vi "Find Repeating Ortho-Subset in GB 2014-12-15.vi"(6 "Presorted?":bool, 8 "Tolerance (A)":dbl=0.5, 9 "Slab Y":dbl=6.0, 10 "Slab X":dbl=6.0, 11 "Grain Boundary":T1={"Structure Name"="CdTe Expanded to Box", "Lattice vector a"=[19.0, 0.0, 0.0], "Lattice vector b"=[0.0, 90.0, 0.0], "Lattice vector c"=[0.0, 0.0, 19.98181818181818], "Atoms Array"=[{"Atom Name"="Cd", "Positions (Direct)"=array501x3[1503 elements], "Positions (Cartesian)"=array501x3[1503 elements]}, {"Atom Name"="Te", "Positions (Direct)"=array504x3[1512 elements], "Positions (Cartesian)"=array504x3[1512 elements]}], "# of atoms"=1005} {"Atoms Array"."Positions (Cartesian)" format="%#_4f"; "Atoms Array"."Positions (Direct)" format="%#_4f"}) -> (0 "Repeating Y Length Scale":dbl=4.670554880088597, 1 "Subset Y found?!":bool, 2 "Repeating X Length Scale":dbl, 3 "Subset X found?!":bool)   [LabVIEW 2010]
uses:
  <vilib>/Analysis/NI_AALPro.lvlib
  <vilib>/Analysis/_algsub.llb/Real Vector Norm.vi
panel:
  out "Array 3":dbl[](array[numeric])
  out "Array 2":dbl[][](array[numeric])
  out "Array":dbl[][](array[numeric])
  out "array w/ subset deleted":dbl[](array[numeric])
  in  "Y index to Search":i32=1
  in  "X index to Search":i32
  out "Length Candidates X":dbl[](array[numeric])=[0.0, 6.615785553057252, 13.231571106114504]
  out "Length Candidates Y":dbl[](array[numeric])=[4.670554880088597, 84.3349903964902, 0.0, 79.6644355164016, -4.670554880088597, 74.993880636313, 70.32332575622439, 65.6527708761358, 60.98221599604721, 56.311661115958614]
  out "Slab":T2(array[cluster])=[{"Atom Name"="Cd", "Positions (Cartesian)"=[[0.0, 4.670554880088597, 0.7469022070093141], [0.0, 0.0, 1.0119047619047619], [0.0, 4.935557434984045, 5.417457087097911], [0.0, 0.2650025548954482, 5.6824596419933595], [0.0, 5.200559989879494, 10.088011967186508], [0.0, 0.5300051097908964, 10.353014522081956], [0.0, 5.465562544774942, 14.758566847275105], [0.0, 0.7950076646863447, 15.023569402170553], [0.0, 5.73056509967039, 19.4291217273637], [0.0, 1.0600102195817929, 19.69412428225915], [3.307892776528626, 2.4677787174920227, 3.2146809245013364], [3.307892776528626, 2.732781272387471, 7.885235804589934], [3.307892776528626, 2.997783827282919, 12.55579068467853], [3.307892776528626, 3.2627863821783674, 17.226345564767126]]}, {"Atom Name"="Te", "Positions (Cartesian)"=[[1.653946388264313, 4.803056157536321, 3.0821796470536116], [1.653946388264313, 0.1325012774477241, 3.3471822019490607], [1.653946388264313, 5.068058712431769, 7.752734527142209], [1.653946388264313, 0.397503832343172, 8.017737082037657], [1.653946388264313, 5.333061267327217, 12.423289407230806], [1.653946388264313, 0.6625063872386205, 12.688291962126254], [1.653946388264313, 5.598063822222666, 17.093844287319403], [1.653946388264313, 0.9275089421340684, 17.358846842214852], [4.96183916479294, 2.3352774400442984, 0.879403484457038], [4.96183916479294, 2.6002799949397466, 5.549958364545636], [4.96183916479294, 2.865282549835195, 10.220513244634233], [4.96183916479294, 3.130285104730643, 14.891068124722828], [4.96183916479294, 3.3952876596260912, 19.561623004811427]]}] {"Positions (Cartesian)" format="%#_4f"}
  out "Supercell without slab":T2(array[cluster])=[{"Atom Name"="Cd", "Positions (Cartesian)"=[0.0, 14.01166464026579, 0.21689709721841766, 0.0, 9.341109760177194, 0.48189965211386543, 0.0, 89.0055452765788, 0.6474110989798403, 0.0, 4.670554880088597, 0.7469022070093141, 0.0, 84.3349903964902, 0.9124136538752889, 0.0, 0.0, 1.0119047619047619, 0.0, 79.6644355164016, 1.1774162087707394, 0.0, 74.993880636313, 1.442418763666188, 0.0, 70.3233257562244, 1.7074213185616385, 0.0, 65.6527708761358, 1.9724238734570871, 0.0, 60.98221599604721, 2.2374264283525305, 0.0, 56.311661115958614, 2.502428983247979, 0.0, 51.64110623587002, 2.7674315381434296, 0.0, 46.97055135578142, 3.0324340930388782, 0.0, 42.29999647569282, 3.297436647934325, 0.0, 37.62944159560422, 3.5624392028297738, 0.0, 32.95888671551563, 3.8274417577252207, 0.0, 28.288331835427034, 4.092444312620669, 0.0, 23.617776955338435, 4.357446867516118, 0.0, 18.947222075249837, 4.622449422411567, 0.0, 14.27666719516124, 4.887451977307014, 0.0, 9.606112315072641, 5.152454532202463, 0.0, 89.27054783147425, 5.317965979068438, 0.0, 4.935557434984045, 5.417457087097911, 0.0, 84.59999295138564, 5.582968533963888, 0.0, 0.2650025548954482, 5.6824596419933595, 0.0, 79.92943807129704, 5.847971088859337, 0.0, 75.25888319120845, 6.1129736437547875, 0.0, 70.58832831111985, 6.377976198650236, 0.0, 65.91777343103126, 6.6429787535456795, 0.0, 61.247218550942655, 6.907981308441128, 0.0, 56.57666367085406, 7.172983863336579, 0.0, 51.906108790765465, 7.437986418232027, 0.0, 47.23555391067687, 7.702988973127474, 0.0, 42.56499903058827, 7.967991528022923, 0.0, 37.89444415049967, 8.23299408291837, 0.0, 33.22388927041108, 8.497996637813818, 0.0, 28.55333439032248, 8.762999192709266, 0.0, 23.882779510233885, 9.028001747604716, 0.0, 19.212224630145286, 9.293004302500165, 0.0, 14.541669750056688, 9.558006857395611, 0.0, 9.87111486996809, 9.82300941229106, 0.0, 89.53555038636969, 9.988520859157038, 0.0, 5.200559989879494, 10.088011967186508, 0.0, 84.86499550628109, 10.253523414052486, 0.0, 0.5300051097908964, 10.353014522081956, 0.0, 80.19444062619249, 10.518525968947937, 0.0, 75.5238857461039, 10.783528523843385, 0.0, 70.85333086601531, 11.04853107873883, 0.0, 66.18277598592671, 11.313533633634277, 0.0, 61.51222110583811, 11.578536188529728, 0.0, 56.841666225749506, 11.843538743425176, 0.0, 52.17111134566091, 12.108541298320624, 0.0, 47.500556465572316, 12.373543853216072, 0.0, 42.83000158548372, 12.63854640811152, 0.0, 38.15944670539512, 12.903548963006967, 0.0, 33.488891825306524, 13.168551517902415, 0.0, 28.81833694521793, 13.433554072797865, 0.0, 24.14778206512933, 13.698556627693314, 0.0, 19.477227185040736, 13.963559182588762, 0.0, 14.806672304952137, 14.22856173748421, 0.0, 10.136117424863539, 14.493564292379657, 0.0, 89.80055294126514, 14.659075739245635, 0.0, 5.465562544774942, 14.758566847275105, 0.0, 85.12999806117654, 14.924078294141086, 0.0, 0.7950076646863447, 15.023569402170553, 0.0, 80.45944318108793, 15.189080849036534, 0.0, 75.78888830099935, 15.454083403931978, 0.0, 71.11833342091076, 15.719085958827426, 0.0, 66.44777854082216, 15.984088513722877, 0.0, 61.777223660733554, 16.249091068618327, 0.0, 57.10666878064496, 16.514093623513773, 0.0, 52.43611390055636, 16.77909617840922, 0.0, 47.76555902046776, 17.04409873330467, 0.0, 43.09500414037917, 17.309101288200118, 0.0, 38.42444926029057, 17.574103843095568, 0.0, 33.75389438020197, 17.839106397991014, 0.0, 29.083339500113375, 18.104108952886463, 0.0, 24.41278462002478, 18.36911150778191, 0.0, 19.74222973993618, 18.63411406267736, 0.0, 15.071674859847585, 18.89911661757281, 0.0, 10.401119979758988, 19.164119172468254, 0.0, 5.73056509967039, 19.4291217273637, 0.0, 85.39500061607198, 19.594633174229685, 0.0, 1.0600102195817929, 19.69412428225915, 0.0, 80.7244457359834, 19.859635729125127, 3.307892776528626, 58.51443727855519, 0.03465026575595598, 3.307892776528626, 53.84388239846659, 0.2996528206514042, 3.307892776528626, 49.173327518377995, 0.5646553755468551, 3.307892776528626, 44.5027726382894, 0.8296579304423033, 3.307892776528626, 39.8322177582008, 1.0946604853377506, 3.307892776528626, 35.161662878112196, 1.3596630402331988, 3.307892776528626, 30.491107998023608, 1.6246655951286462, 3.307892776528626, 25.82055311793501, 1.8896681500240944, 3.307892776528626, 21.14999823784641, 2.1546707049195435, 3.307892776528626, 16.479443357757813, 2.4196732598149917, 3.307892776528626, 11.808888477669216, 2.68467581471044, 3.307892776528626, 7.138333597580619, 2.949678369605888, 3.307892776528626, 86.80276911398222, 3.115189816471863, 3.307892776528626, 2.4677787174920227, 3.2146809245013364, 3.307892776528626, 82.13221423389362, 3.380192371367314, 3.307892776528626, 77.46165935380502, 3.645194926262762, 3.307892776528626, 72.79110447371643, 3.910197481158213, 3.307892776528626, 68.12054959362783, 4.175200036053662, 3.307892776528626, 63.44999471353923, 4.440202590949105, 3.307892776528626, 58.77943983345064, 4.705205145844554, 3.307892776528626, 54.10888495336204, 4.970207700740004, 3.307892776528626, 49.43833007327345, 5.235210255635453, 3.307892776528626, 44.767775193184846, 5.5002128105309, 3.307892776528626, 40.097220313096244, 5.765215365426348, 3.307892776528626, 35.426665433007656, 6.030217920321795, 3.307892776528626, 30.756110552919058, 6.295220475217244, 3.307892776528626, 26.08555567283046, 6.5602230301126925, 3.307892776528626, 21.41500079274186, 6.825225585008141, 3.307892776528626, 16.744445912653262, 7.090228139903589, 3.307892776528626, 12.073891032564665, 7.355230694799037, 3.307892776528626, 7.403336152476069, 7.620233249694485, 3.307892776528626, 87.06777166887767, 7.785744696560463, 3.307892776528626, 2.732781272387471, 7.885235804589934, 3.307892776528626, 82.39721678878907, 8.050747251455912, 3.307892776528626, 77.72666190870048, 8.315749806351363, 3.307892776528626, 73.05610702861188, 8.58075236124681, 3.307892776528626, 68.38555214852329, 8.845754916142255, 3.307892776528626, 63.714997268434686, 9.110757471037703, 3.307892776528626, 59.044442388346084, 9.375760025933154, 3.307892776528626, 54.37388750825748, 9.640762580828602, 3.307892776528626, 49.703332628168894, 9.90576513572405, 3.307892776528626, 45.03277774808029, 10.170767690619497, 3.307892776528626, 40.3622228679917, 10.435770245514945, 3.307892776528626, 35.6916679879031, 10.700772800410393, 3.307892776528626, 31.021113107814504, 10.96577535530584, 3.307892776528626, 26.350558227725905, 11.23077791020129, 3.307892776528626, 21.68000334763731, 11.49578046509674, 3.307892776528626, 17.00944846754871, 11.760783019992187, 3.307892776528626, 12.338893587460113, 12.025785574887635, 3.307892776528626, 7.668338707371516, 12.290788129783083, 3.307892776528626, 87.33277422377311, 12.45629957664906, 3.307892776528626, 2.997783827282919, 12.55579068467853, 3.307892776528626, 82.66221934368451, 12.721302131544512, 3.307892776528626, 77.99166446359591, 12.98630468643996, 3.307892776528626, 73.32110958350734, 13.251307241335404, 3.307892776528626, 68.65055470341873, 13.516309796230852, 3.307892776528626, 63.97999982333013, 13.781312351126303, 3.307892776528626, 59.30944494324153, 14.04631490602175, 3.307892776528626, 54.638890063152935, 14.311317460917198, 3.307892776528626, 49.96833518306434, 14.576320015812646, 3.307892776528626, 45.297780302975745, 14.841322570708094, 3.307892776528626, 40.62722542288715, 15.106325125603542, 3.307892776528626, 35.95667054279855, 15.37132768049899, 3.307892776528626, 31.28611566270995, 15.63633023539444, 3.307892776528626, 26.615560782621355, 15.901332790289889, 3.307892776528626, 21.945005902532756, 16.166335345185335, 3.307892776528626, 17.27445102244416, 16.431337900080784, 3.307892776528626, 12.603896142355563, 16.69634045497623, 3.307892776528626, 7.933341262266964, 16.96134300987168, 3.307892776528626, 87.59777677866856, 17.12685445673766, 3.307892776528626, 3.2627863821783674, 17.226345564767126, 3.307892776528626, 82.92722189857996, 17.391857011633107, 3.307892776528626, 78.25666701849137, 17.656859566528553, 3.307892776528626, 73.58611213840277, 17.921862121424, 3.307892776528626, 68.91555725831418, 18.186864676319452, 3.307892776528626, 64.24500237822558, 18.451867231214898, 3.307892776528626, 59.57444749813698, 18.716869786110347, 3.307892776528626, 54.90389261804839, 18.981872341005793, 3.307892776528626, 50.233337737959786, 19.246874895901243, 3.307892776528626, 45.562782857871184, 19.51187745079669, 3.307892776528626, 40.892227977782596, 19.776880005692142, 6.615785553057252, 14.01166464026579, 0.21689709721841766, 6.615785553057252, 9.341109760177194, 0.48189965211386543, 6.615785553057252, 89.0055452765788, 0.6474110989798403, 6.615785553057252, 4.670554880088597, 0.7469022070093141, 6.615785553057252, 84.3349903964902, 0.9124136538752889, 6.615785553057252, 0.0, 1.0119047619047619, 6.615785553057252, 79.6644355164016, 1.1774162087707394, 6.615785553057252, 74.993880636313, 1.442418763666188, 6.615785553057252, 70.3233257562244, 1.7074213185616385, 6.615785553057252, 65.6527708761358, 1.9724238734570871, 6.615785553057252, 60.98221599604721, 2.2374264283525305, 6.615785553057252, 56.311661115958614, 2.502428983247979, 6.615785553057252, 51.64110623587002, 2.7674315381434296, 6.615785553057252, 46.97055135578142, 3.0324340930388782, 6.615785553057252, 42.29999647569282, 3.297436647934325, 6.615785553057252, 37.62944159560422, 3.5624392028297738, 6.615785553057252, 32.95888671551563, 3.8274417577252207, 6.615785553057252, 28.288331835427034, 4.092444312620669, 6.615785553057252, 23.617776955338435, 4.357446867516118, 6.615785553057252, 18.947222075249837, 4.622449422411567, 6.615785553057252, 14.27666719516124, 4.887451977307014, 6.615785553057252, 9.606112315072641, 5.152454532202463, 6.615785553057252, 89.27054783147425, 5.317965979068438, 6.615785553057252, 4.935557434984045, 5.417457087097911, 6.615785553057252, 84.59999295138564, 5.582968533963888, 6.615785553057252, 0.2650025548954482, 5.6824596419933595, 6.615785553057252, 79.92943807129704, 5.847971088859337, 6.615785553057252, 75.25888319120845, 6.1129736437547875, 6.615785553057252, 70.58832831111985, 6.377976198650236, 6.615785553057252, 65.91777343103126, 6.6429787535456795, 6.615785553057252, 61.247218550942655, 6.907981308441128, 6.615785553057252, 56.57666367085406, 7.172983863336579, 6.615785553057252, 51.906108790765465, 7.437986418232027, 6.615785553057252, 47.23555391067687, 7.702988973127474, 6.615785553057252, 42.56499903058827, 7.967991528022923, 6.615785553057252, 37.89444415049967, 8.23299408291837, 6.615785553057252, 33.22388927041108, 8.497996637813818, 6.615785553057252, 28.55333439032248, 8.762999192709266, 6.615785553057252, 23.882779510233885, 9.028001747604716, 6.615785553057252, 19.212224630145286, 9.293004302500165, 6.615785553057252, 14.541669750056688, 9.558006857395611, 6.615785553057252, 9.87111486996809, 9.82300941229106, 6.615785553057252, 89.53555038636969, 9.988520859157038, 6.615785553057252, 5.200559989879494, 10.088011967186508, 6.615785553057252, 84.86499550628109, 10.253523414052486, 6.615785553057252, 0.5300051097908964, 10.353014522081956, 6.615785553057252, 80.19444062619249, 10.518525968947937, 6.615785553057252, 75.5238857461039, 10.783528523843385, 6.615785553057252, 70.85333086601531, 11.04853107873883, 6.615785553057252, 66.18277598592671, 11.313533633634277, 6.615785553057252, 61.51222110583811, 11.578536188529728, 6.615785553057252, 56.841666225749506, 11.843538743425176, 6.615785553057252, 52.17111134566091, 12.108541298320624, 6.615785553057252, 47.500556465572316, 12.373543853216072, 6.615785553057252, 42.83000158548372, 12.63854640811152, 6.615785553057252, 38.15944670539512, 12.903548963006967, 6.615785553057252, 33.488891825306524, 13.168551517902415, 6.615785553057252, 28.81833694521793, 13.433554072797865, 6.615785553057252, 24.14778206512933, 13.698556627693314, 6.615785553057252, 19.477227185040736, 13.963559182588762, 6.615785553057252, 14.806672304952137, 14.22856173748421, 6.615785553057252, 10.136117424863539, 14.493564292379657, 6.615785553057252, 89.80055294126514, 14.659075739245635, 6.615785553057252, 5.465562544774942, 14.758566847275105, 6.615785553057252, 85.12999806117654, 14.924078294141086, 6.615785553057252, 0.7950076646863447, 15.023569402170553, 6.615785553057252, 80.45944318108793, 15.189080849036534, 6.615785553057252, 75.78888830099935, 15.454083403931978, 6.615785553057252, 71.11833342091076, 15.719085958827426, 6.615785553057252, 66.44777854082216, 15.984088513722877, 6.615785553057252, 61.777223660733554, 16.249091068618327, 6.615785553057252, 57.10666878064496, 16.514093623513773, 6.615785553057252, 52.43611390055636, 16.77909617840922, 6.615785553057252, 47.76555902046776, 17.04409873330467, 6.615785553057252, 43.09500414037917, 17.309101288200118, 6.615785553057252, 38.42444926029057, 17.574103843095568, 6.615785553057252, 33.75389438020197, 17.839106397991014, 6.615785553057252, 29.083339500113375, 18.104108952886463, 6.615785553057252, 24.41278462002478, 18.36911150778191, 6.615785553057252, 19.74222973993618, 18.63411406267736, 6.615785553057252, 15.071674859847585, 18.89911661757281, 6.615785553057252, 10.401119979758988, 19.164119172468254, 6.615785553057252, 5.73056509967039, 19.4291217273637, 6.615785553057252, 85.39500061607198, 19.594633174229685, 6.615785553057252, 1.0600102195817929, 19.69412428225915, 6.615785553057252, 80.7244457359834, 19.859635729125127, 9.92367832958588, 58.51443727855519, 0.03465026575595598, 9.92367832958588, 53.84388239846659, 0.2996528206514042, 9.92367832958588, 49.173327518377995, 0.5646553755468551, 9.92367832958588, 44.5027726382894, 0.8296579304423033, 9.92367832958588, 39.8322177582008, 1.0946604853377506, 9.92367832958588, 35.161662878112196, 1.3596630402331988, 9.92367832958588, 30.491107998023608, 1.6246655951286462, 9.92367832958588, 25.82055311793501, 1.8896681500240944, 9.92367832958588, 21.14999823784641, 2.1546707049195435, 9.92367832958588, 16.479443357757813, 2.4196732598149917, 9.92367832958588, 11.808888477669216, 2.68467581471044, 9.92367832958588, 7.138333597580619, 2.949678369605888, 9.92367832958588, 86.80276911398222, 3.115189816471863, 9.92367832958588, 2.4677787174920227, 3.2146809245013364, 9.92367832958588, 82.13221423389362, 3.380192371367314, 9.92367832958588, 77.46165935380502, 3.645194926262762, 9.92367832958588, 72.79110447371643, 3.910197481158213, 9.92367832958588, 68.12054959362783, 4.175200036053662, 9.92367832958588, 63.44999471353923, 4.440202590949105, 9.92367832958588, 58.77943983345064, 4.705205145844554, 9.92367832958588, 54.10888495336204, 4.970207700740004, 9.92367832958588, 49.43833007327345, 5.235210255635453, 9.92367832958588, 44.767775193184846, 5.5002128105309, 9.92367832958588, 40.097220313096244, 5.765215365426348, 9.92367832958588, 35.426665433007656, 6.030217920321795, 9.92367832958588, 30.756110552919058, 6.295220475217244, 9.92367832958588, 26.08555567283046, 6.5602230301126925, 9.92367832958588, 21.41500079274186, 6.825225585008141, 9.92367832958588, 16.744445912653262, 7.090228139903589, 9.92367832958588, 12.073891032564665, 7.355230694799037, 9.92367832958588, 7.403336152476069, 7.620233249694485, 9.92367832958588, 87.06777166887767, 7.785744696560463, 9.92367832958588, 2.732781272387471, 7.885235804589934, 9.92367832958588, 82.39721678878907, 8.050747251455912, 9.92367832958588, 77.72666190870048, 8.315749806351363, 9.92367832958588, 73.05610702861188, 8.58075236124681, 9.92367832958588, 68.38555214852329, 8.845754916142255, 9.92367832958588, 63.714997268434686, 9.110757471037703, 9.92367832958588, 59.044442388346084, 9.375760025933154, 9.92367832958588, 54.37388750825748, 9.640762580828602, 9.92367832958588, 49.703332628168894, 9.90576513572405, 9.92367832958588, 45.03277774808029, 10.170767690619497, 9.92367832958588, 40.3622228679917, 10.435770245514945, 9.92367832958588, 35.6916679879031, 10.700772800410393, 9.92367832958588, 31.021113107814504, 10.96577535530584, 9.92367832958588, 26.350558227725905, 11.23077791020129, 9.92367832958588, 21.68000334763731, 11.49578046509674, 9.92367832958588, 17.00944846754871, 11.760783019992187, 9.92367832958588, 12.338893587460113, 12.025785574887635, 9.92367832958588, 7.668338707371516, 12.290788129783083, 9.92367832958588, 87.33277422377311, 12.45629957664906, 9.92367832958588, 2.997783827282919, 12.55579068467853, 9.92367832958588, 82.66221934368451, 12.721302131544512, 9.92367832958588, 77.99166446359591, 12.98630468643996, 9.92367832958588, 73.32110958350734, 13.251307241335404, 9.92367832958588, 68.65055470341873, 13.516309796230852, 9.92367832958588, 63.97999982333013, 13.781312351126303, 9.92367832958588, 59.30944494324153, 14.04631490602175, 9.92367832958588, 54.638890063152935, 14.311317460917198, 9.92367832958588, 49.96833518306434, 14.576320015812646, 9.92367832958588, 45.297780302975745, 14.841322570708094, 9.92367832958588, 40.62722542288715, 15.106325125603542, 9.92367832958588, 35.95667054279855, 15.37132768049899, 9.92367832958588, 31.28611566270995, 15.63633023539444, 9.92367832958588, 26.615560782621355, 15.901332790289889, 9.92367832958588, 21.945005902532756, 16.166335345185335, 9.92367832958588, 17.27445102244416, 16.431337900080784, 9.92367832958588, 12.603896142355563, 16.69634045497623, 9.92367832958588, 7.933341262266964, 16.96134300987168, 9.92367832958588, 87.59777677866856, 17.12685445673766, 9.92367832958588, 3.2627863821783674, 17.226345564767126, 9.92367832958588, 82.92722189857996, 17.391857011633107, 9.92367832958588, 78.25666701849137, 17.656859566528553, 9.92367832958588, 73.58611213840277, 17.921862121424, 9.92367832958588, 68.91555725831418, 18.186864676319452, 9.92367832958588, 64.24500237822558, 18.451867231214898, 9.92367832958588, 59.57444749813698, 18.716869786110347, 9.92367832958588, 54.90389261804839, 18.981872341005793, 9.92367832958588, 50.233337737959786, 19.246874895901243, 9.92367832958588, 45.562782857871184, 19.51187745079669, 9.92367832958588, 40.892227977782596, 19.776880005692142, 13.231571106114504, 14.01166464026579, 0.21689709721841766, 13.231571106114504, 9.341109760177194, 0.48189965211386543, 13.231571106114504, 89.0055452765788, 0.6474110989798403, 13.231571106114504, 4.670554880088597, 0.7469022070093141, 13.231571106114504, 84.3349903964902, 0.9124136538752889, 13.231571106114504, 0.0, 1.0119047619047619, 13.231571106114504, 79.6644355164016, 1.1774162087707394, 13.231571106114504, 74.993880636313, 1.442418763666188, 13.231571106114504, 70.3233257562244, 1.7074213185616385, 13.231571106114504, 65.6527708761358, 1.9724238734570871, 13.231571106114504, 60.98221599604721, 2.2374264283525305, 13.231571106114504, 56.311661115958614, 2.502428983247979, 13.231571106114504, 51.64110623587002, 2.7674315381434296, 13.231571106114504, 46.97055135578142, 3.0324340930388782, 13.231571106114504, 42.29999647569282, 3.297436647934325, 13.231571106114504, 37.62944159560422, 3.5624392028297738, 13.231571106114504, 32.95888671551563, 3.8274417577252207, 13.231571106114504, 28.288331835427034, 4.092444312620669, 13.231571106114504, 23.617776955338435, 4.357446867516118, 13.231571106114504, 18.947222075249837, 4.622449422411567, 13.231571106114504, 14.27666719516124, 4.887451977307014, 13.231571106114504, 9.606112315072641, 5.152454532202463, 13.231571106114504, 89.27054783147425, 5.317965979068438, 13.231571106114504, 4.935557434984045, 5.417457087097911, 13.231571106114504, 84.59999295138564, 5.582968533963888, 13.231571106114504, 0.2650025548954482, 5.6824596419933595, 13.231571106114504, 79.92943807129704, 5.847971088859337, 13.231571106114504, 75.25888319120845, 6.1129736437547875, 13.231571106114504, 70.58832831111985, 6.377976198650236, 13.231571106114504, 65.91777343103126, 6.6429787535456795, 13.231571106114504, 61.247218550942655, 6.907981308441128, 13.231571106114504, 56.57666367085406, 7.172983863336579, 13.231571106114504, 51.906108790765465, 7.437986418232027, 13.231571106114504, 47.23555391067687, 7.702988973127474, 13.231571106114504, 42.56499903058827, 7.967991528022923, 13.231571106114504, 37.89444415049967, 8.23299408291837, 13.231571106114504, 33.22388927041108, 8.497996637813818, 13.231571106114504, 28.55333439032248, 8.762999192709266, 13.231571106114504, 23.882779510233885, 9.028001747604716, 13.231571106114504, 19.212224630145286, 9.293004302500165, 13.231571106114504, 14.541669750056688, 9.558006857395611, 13.231571106114504, 9.87111486996809, 9.82300941229106, 13.231571106114504, 89.53555038636969, 9.988520859157038, 13.231571106114504, 5.200559989879494, 10.088011967186508, 13.231571106114504, 84.86499550628109, 10.253523414052486, 13.231571106114504, 0.5300051097908964, 10.353014522081956, 13.231571106114504, 80.19444062619249, 10.518525968947937, 13.231571106114504, 75.5238857461039, 10.783528523843385, 13.231571106114504, 70.85333086601531, 11.04853107873883, 13.231571106114504, 66.18277598592671, 11.313533633634277, 13.231571106114504, 61.51222110583811, 11.578536188529728, 13.231571106114504, 56.841666225749506, 11.843538743425176, 13.231571106114504, 52.17111134566091, 12.108541298320624, 13.231571106114504, 47.500556465572316, 12.373543853216072, 13.231571106114504, 42.83000158548372, 12.63854640811152, 13.231571106114504, 38.15944670539512, 12.903548963006967, 13.231571106114504, 33.488891825306524, 13.168551517902415, 13.231571106114504, 28.81833694521793, 13.433554072797865, 13.231571106114504, 24.14778206512933, 13.698556627693314, 13.231571106114504, 19.477227185040736, 13.963559182588762, 13.231571106114504, 14.806672304952137, 14.22856173748421, 13.231571106114504, 10.136117424863539, 14.493564292379657, 13.231571106114504, 89.80055294126514, 14.659075739245635, 13.231571106114504, 5.465562544774942, 14.758566847275105, 13.231571106114504, 85.12999806117654, 14.924078294141086, 13.231571106114504, 0.7950076646863447, 15.023569402170553, 13.231571106114504, 80.45944318108793, 15.189080849036534, 13.231571106114504, 75.78888830099935, 15.454083403931978, 13.231571106114504, 71.11833342091076, 15.719085958827426, 13.231571106114504, 66.44777854082216, 15.984088513722877, 13.231571106114504, 61.777223660733554, 16.249091068618327, 13.231571106114504, 57.10666878064496, 16.514093623513773, 13.231571106114504, 52.43611390055636, 16.77909617840922, 13.231571106114504, 47.76555902046776, 17.04409873330467, 13.231571106114504, 43.09500414037917, 17.309101288200118, 13.231571106114504, 38.42444926029057, 17.574103843095568, 13.231571106114504, 33.75389438020197, 17.839106397991014, 13.231571106114504, 29.083339500113375, 18.104108952886463, 13.231571106114504, 24.41278462002478, 18.36911150778191, 13.231571106114504, 19.74222973993618, 18.63411406267736, 13.231571106114504, 15.071674859847585, 18.89911661757281, 13.231571106114504, 10.401119979758988, 19.164119172468254, 13.231571106114504, 5.73056509967039, 19.4291217273637, 13.231571106114504, 85.39500061607198, 19.594633174229685, 13.231571106114504, 1.0600102195817929, 19.69412428225915, 13.231571106114504, 80.7244457359834, 19.859635729125127, 16.53946388264313, 58.51443727855519, 0.03465026575595598, 16.53946388264313, 53.84388239846659, 0.2996528206514042, 16.53946388264313, 49.173327518377995, 0.5646553755468551, 16.53946388264313, 44.5027726382894, 0.8296579304423033, 16.53946388264313, 39.8322177582008, 1.0946604853377506, 16.53946388264313, 35.161662878112196, 1.3596630402331988, 16.53946388264313, 30.491107998023608, 1.6246655951286462, 16.53946388264313, 25.82055311793501, 1.8896681500240944, 16.53946388264313, 21.14999823784641, 2.1546707049195435, 16.53946388264313, 16.479443357757813, 2.4196732598149917, 16.53946388264313, 11.808888477669216, 2.68467581471044, 16.53946388264313, 7.138333597580619, 2.949678369605888, 16.53946388264313, 86.80276911398222, 3.115189816471863, 16.53946388264313, 2.4677787174920227, 3.2146809245013364, 16.53946388264313, 82.13221423389362, 3.380192371367314, 16.53946388264313, 77.46165935380502, 3.645194926262762, 16.53946388264313, 72.79110447371643, 3.910197481158213, 16.53946388264313, 68.12054959362783, 4.175200036053662, 16.53946388264313, 63.44999471353923, 4.440202590949105, 16.53946388264313, 58.77943983345064, 4.705205145844554, 16.53946388264313, 54.10888495336204, 4.970207700740004, 16.53946388264313, 49.43833007327345, 5.235210255635453, 16.53946388264313, 44.767775193184846, 5.5002128105309, 16.53946388264313, 40.097220313096244, 5.765215365426348, 16.53946388264313, 35.426665433007656, 6.030217920321795, 16.53946388264313, 30.756110552919058, 6.295220475217244, 16.53946388264313, 26.08555567283046, 6.5602230301126925, 16.53946388264313, 21.41500079274186, 6.825225585008141, 16.53946388264313, 16.744445912653262, 7.090228139903589, 16.53946388264313, 12.073891032564665, 7.355230694799037, 16.53946388264313, 7.403336152476069, 7.620233249694485, 16.53946388264313, 87.06777166887767, 7.785744696560463, 16.53946388264313, 2.732781272387471, 7.885235804589934, 16.53946388264313, 82.39721678878907, 8.050747251455912, 16.53946388264313, 77.72666190870048, 8.315749806351363, 16.53946388264313, 73.05610702861188, 8.58075236124681, 16.53946388264313, 68.38555214852329, 8.845754916142255, 16.53946388264313, 63.714997268434686, 9.110757471037703, 16.53946388264313, 59.044442388346084, 9.375760025933154, 16.53946388264313, 54.37388750825748, 9.640762580828602, 16.53946388264313, 49.703332628168894, 9.90576513572405, 16.53946388264313, 45.03277774808029, 10.170767690619497, 16.53946388264313, 40.3622228679917, 10.435770245514945, 16.53946388264313, 35.6916679879031, 10.700772800410393, 16.53946388264313, 31.021113107814504, 10.96577535530584, 16.53946388264313, 26.350558227725905, 11.23077791020129, 16.53946388264313, 21.68000334763731, 11.49578046509674, 16.53946388264313, 17.00944846754871, 11.760783019992187, 16.53946388264313, 12.338893587460113, 12.025785574887635, 16.53946388264313, 7.668338707371516, 12.290788129783083, 16.53946388264313, 87.33277422377311, 12.45629957664906, 16.53946388264313, 2.997783827282919, 12.55579068467853, 16.53946388264313, 82.66221934368451, 12.721302131544512, 16.53946388264313, 77.99166446359591, 12.98630468643996, 16.53946388264313, 73.32110958350734, 13.251307241335404, 16.53946388264313, 68.65055470341873, 13.516309796230852, 16.53946388264313, 63.97999982333013, 13.781312351126303, 16.53946388264313, 59.30944494324153, 14.04631490602175, 16.53946388264313, 54.638890063152935, 14.311317460917198, 16.53946388264313, 49.96833518306434, 14.576320015812646, 16.53946388264313, 45.297780302975745, 14.841322570708094, 16.53946388264313, 40.62722542288715, 15.106325125603542, 16.53946388264313, 35.95667054279855, 15.37132768049899, 16.53946388264313, 31.28611566270995, 15.63633023539444, 16.53946388264313, 26.615560782621355, 15.901332790289889, 16.53946388264313, 21.945005902532756, 16.166335345185335, 16.53946388264313, 17.27445102244416, 16.431337900080784, 16.53946388264313, 12.603896142355563, 16.69634045497623, 16.53946388264313, 7.933341262266964, 16.96134300987168, 16.53946388264313, 87.59777677866856, 17.12685445673766, 16.53946388264313, 3.2627863821783674, 17.226345564767126, 16.53946388264313, 82.92722189857996, 17.391857011633107, 16.53946388264313, 78.25666701849137, 17.656859566528553, 16.53946388264313, 73.58611213840277, 17.921862121424, 16.53946388264313, 68.91555725831418, 18.186864676319452, 16.53946388264313, 64.24500237822558, 18.451867231214898, 16.53946388264313, 59.57444749813698, 18.716869786110347, 16.53946388264313, 54.90389261804839, 18.981872341005793, 16.53946388264313, 50.233337737959786, 19.246874895901243, 16.53946388264313, 45.562782857871184, 19.51187745079669, 16.53946388264313, 40.892227977782596, 19.776880005692142]}, ...(2 in all)] {"Positions (Cartesian)" format="%#_4f"}
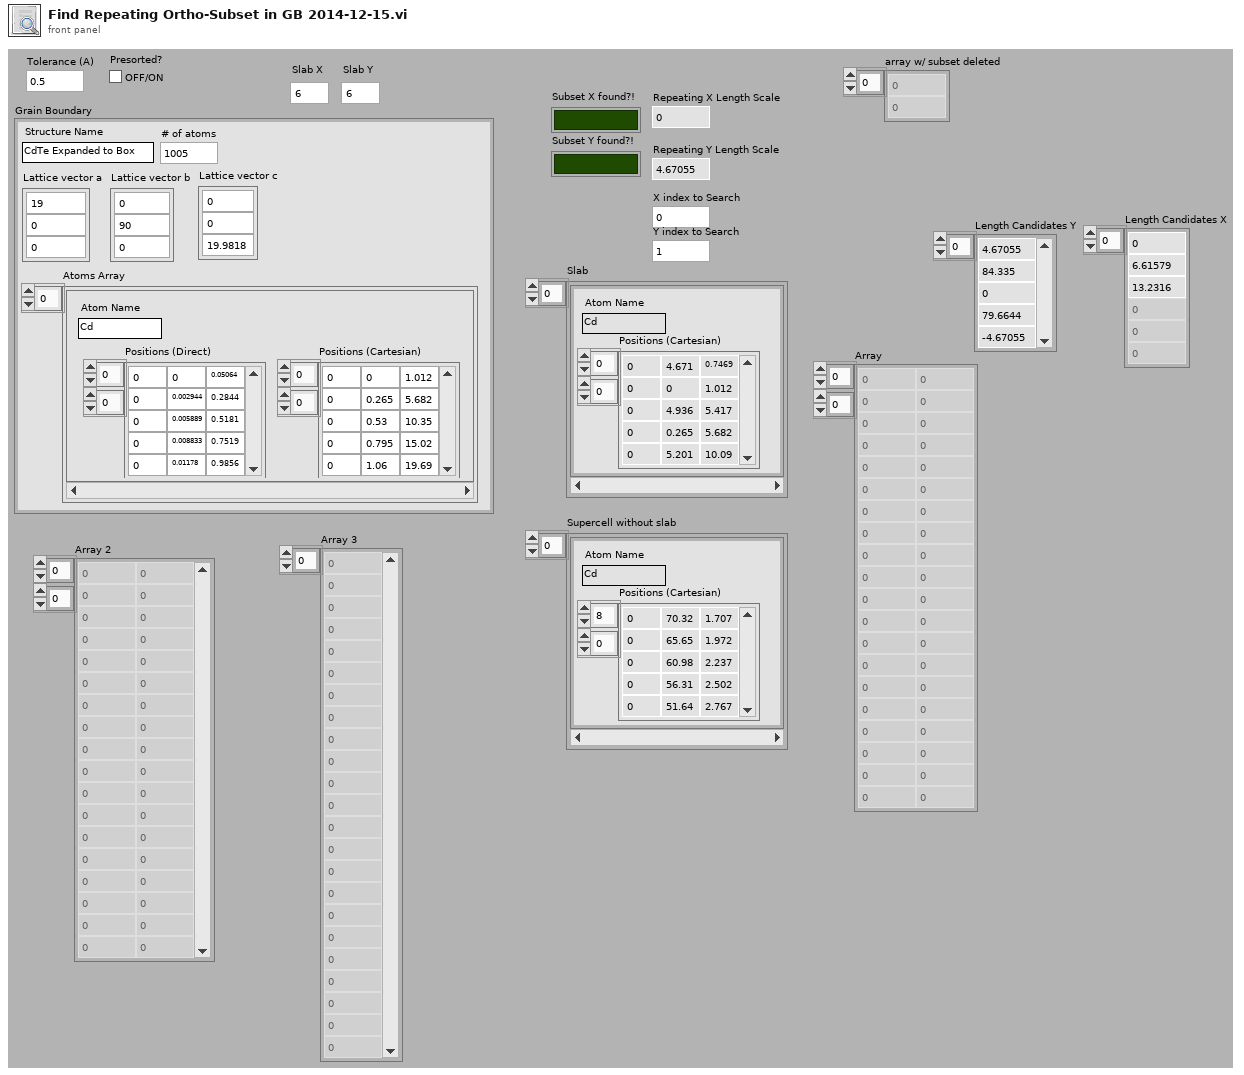
[diagram p1: front panel]
types:
  T1 = cluster{"Structure Name":string, "Lattice vector a":dbl[], "Lattice vector b":dbl[], "Lattice vector c":dbl[], "Atoms Array":cluster{"Atom Name":string, "Positions (Direct)":dbl[][], "Positions (Cartesian)":dbl[][]}[], "# of atoms":i32}
  T2 = cluster{"Atom Name":string, "Positions (Cartesian)":dbl[][]}[]
  T3 = cluster{"Atom Name":string, "Positions (Direct)":dbl[][], "Positions (Cartesian)":dbl[][]}[]
  T4 = cluster{"Atom Name":string, "Output Array":dbl[][]}
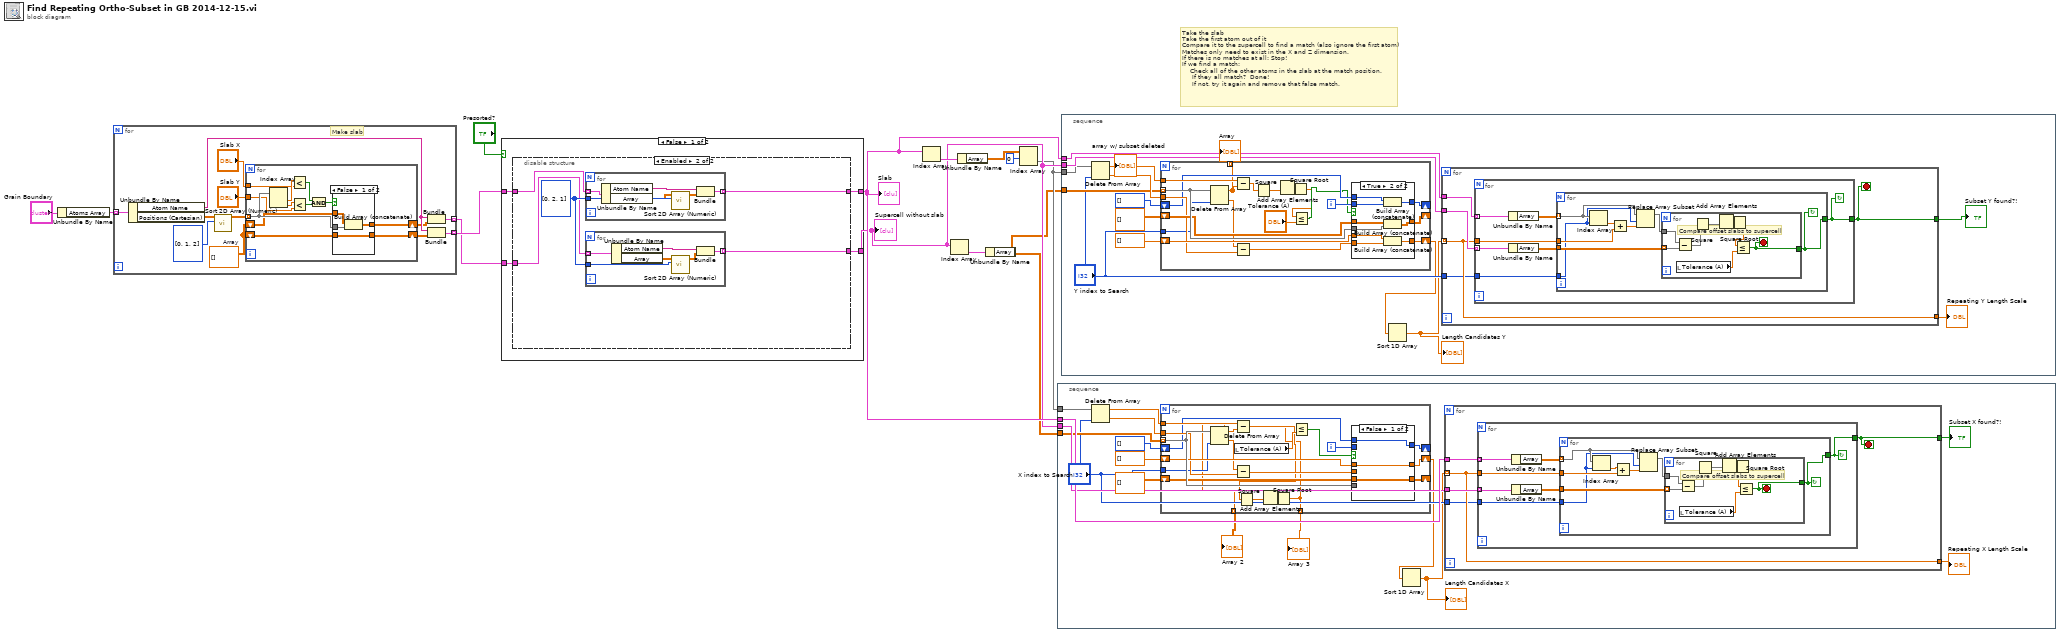
[diagram p0: block diagram]
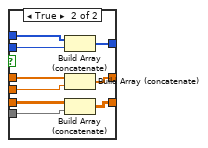
[diagram p3: hidden frame]
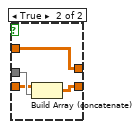
[diagram p4: hidden frame]
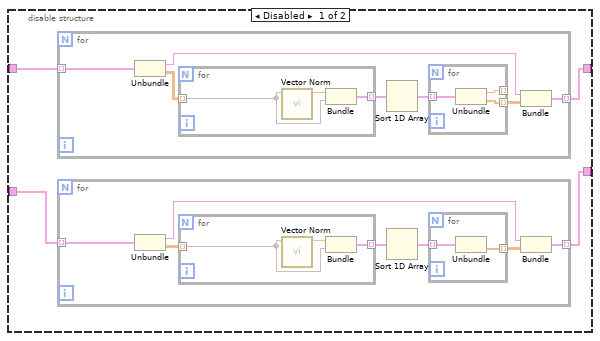
[diagram p5: hidden frame]
diagram:
  # "Take the slab\nTake the first atom out of it\nCompare it to the supercell to find a match (also ignore the first atom)\nMatches only need to exist in the X and Z dimension.\nIf there is no matches at all: Stop!\nIf we find a match: \n    Check all of the other atoms in the slab at the match position.\n     If they all match?  Done!\n     If not, try it again and remove that false match."
  n1 = Unbundle By Name("Grain Boundary") -> ("Atoms Array"=w8:T3)
  n2 = for {
    tunnel: w8 -> [w25] mode=indexing
    tunnel: [w22] -> w6 mode=indexing
    tunnel: [w16] -> w5 mode=indexing
    w15 = dbl[][] []  # Array
    # "Make slab"
    n3 = Unbundle By Name(w25) -> ("Atom Name"=w17:string, "Positions (Cartesian)"=w19:dbl[][])
    n4 = call "Sort 2D Array (Numeric).vi"("Sort by Cols"=i32[] [0, 1, 2], "Input Array"=w19) -> ("Output Array"=w18:dbl[][])  [unwired: 9 in]
    n5 = for {
      tunnel: w18 -> [w35] mode=indexing
      shift-right: [w37] -> w20
      shift-left: w15 -> [w36]
      tunnel: "Slab X" -> [w33]
      tunnel: "Slab Y" -> [w31]
      shift-right: [w27] -> w14
      shift-left: w15 -> [w26]
      n6 = Index Array(array=w35) -> (element #1=w34:dbl, element #2=w32:dbl)  [unwired: 2 in]
      n7 = Less?(x=w34, y=w33) -> (x < y?=w30:bool)
      n8 = Less?(x=w32, y=w31) -> (x < y?=w29:bool)
      n9 = And(x=w30, y=w29) -> (x .and. y?=w28:bool)
      n10 = case shown="False" w28 {
        tunnel: w35 -> [w40 w45]
        tunnel: [w41 w44] -> w37
        tunnel: w36 -> [w41 w43]
        tunnel: [w39 w42] -> w27
        tunnel: w26 -> [w38 w42]
        frame False {
          n11 = Build Array (concatenate)(w38, w40) -> (w39:dbl[][])
        }
        frame True {
          n12 = Build Array (concatenate)(w43, w45) -> (w44:dbl[][])
        }
      }
    }
    n13 = Bundle("Atom Name"=w17, "Array"=w14) -> (w16:cluster{"Atom Name":string, "Array":dbl[][]})  [unwired: 1 in]
    n14 = Bundle("Atom Name"=w17, "Array"=w20) -> (w22:cluster{"Atom Name":string, "Array":dbl[][]})  [unwired: 1 in]
  }
  n15 = case shown="False" "Presorted?" {
    tunnel: w6 -> [w49 w96]
    tunnel: w5 -> [w48 w97]
    tunnel: [w46 w96] -> w4
    tunnel: [w47 w97] -> w3
    frame False {
      n16 = disable-structure shown="Enabled" {
        disable-tunnel: w49 -> [w53 w83]
        disable-tunnel: w48 -> [w52 w80]
        disable-tunnel: [w51 w79] -> w47
        disable-tunnel: [w50 w82] -> w46
        frame Disabled {
          n17 = for {
            tunnel: w53 -> [w72] mode=indexing
            tunnel: [w67] -> w50 mode=indexing
            n18 = Unbundle(w72) -> ("Atom Name"=w68:string, "Array"=w71:dbl[][])
            n19 = for {
              tunnel: w71 -> [w77] mode=indexing
              tunnel: [w76] -> w70 mode=indexing
              n20 = call-poly <vilib>:"Vector Norm.vi"("Input Vector"=w77) -> ("norm"=w78:dbl)  [unwired: 9 in, 1 out]
              n21 = Bundle("norm"=w78, "Array"=w77) -> (w76:cluster{"norm":dbl, "Array":dbl[]})  [unwired: 1 in]
            }
            n22 = Sort 1D Array(array=w70) -> (sorted array=w69:cluster{"norm":dbl, "Array":dbl[]}[])
            n23 = for {
              tunnel: w69 -> [w75] mode=indexing
              tunnel: [w74] -> w66 mode=indexing
              tunnel: [w73] -> _ mode=indexing
              n24 = Unbundle(w75) -> ("norm"=w73:dbl, "Array"=w74:dbl[])
            }
            n25 = Bundle("Atom Name"=w68, "Array"=w66) -> (w67:cluster{"Atom Name":string, "Array":dbl[][]})  [unwired: 1 in]
          }
          n26 = for {
            tunnel: w52 -> [w60] mode=indexing
            tunnel: [w54] -> w51 mode=indexing
            n27 = Unbundle(w60) -> ("Atom Name"=w56:string, "Array"=w59:dbl[][])
            n28 = for {
              tunnel: w59 -> [w64] mode=indexing
              tunnel: [w63] -> w58 mode=indexing
              n29 = call-poly <vilib>:"Vector Norm.vi"("Input Vector"=w64) -> ("norm"=w65:dbl)  [unwired: 9 in, 1 out]
              n30 = Bundle("norm"=w65, "Array"=w64) -> (w63:cluster{"norm":dbl, "Array":dbl[]})  [unwired: 1 in]
            }
            n31 = Sort 1D Array(array=w58) -> (sorted array=w57:cluster{"norm":dbl, "Array":dbl[]}[])
            n32 = for {
              tunnel: w57 -> [w62] mode=indexing
              tunnel: [w61] -> w55 mode=indexing
              n33 = Unbundle(w62) -> ("Array"=w61:dbl[])  [unwired: 1 out]
            }
            n34 = Bundle("Atom Name"=w56, "Array"=w55) -> (w54:cluster{"Atom Name":string, "Array":dbl[][]})  [unwired: 1 in]
          }
        }
        frame Enabled {
          w81 = i32[] [0, 2, 1] ("Sort by Cols")
          n35 = for {
            tunnel: w83 -> [w92] mode=indexing
            tunnel: w81 -> [w95]
            tunnel: [w93] -> w82 mode=indexing
            n36 = Unbundle By Name(w92) -> ("Atom Name"=w91:string, "Array"=w90:dbl[][])
            n37 = call "Sort 2D Array (Numeric).vi"("Sort by Cols"=w95, "Input Array"=w90) -> ("Output Array"=w94:dbl[][])  [unwired: 9 in]
            n38 = Bundle("Atom Name"=w91, "Output Array"=w94) -> (w93:T4)  [unwired: 1 in]
          }
          n39 = for {
            tunnel: w80 -> [w89] mode=indexing
            tunnel: w81 -> [w87]
            tunnel: [w84] -> w79 mode=indexing
            n40 = Unbundle By Name(w89) -> ("Atom Name"=w86:string, "Array"=w88:dbl[][])
            n41 = call "Sort 2D Array (Numeric).vi"("Sort by Cols"=w87, "Input Array"=w88) -> ("Output Array"=w85:dbl[][])  [unwired: 9 in]
            n42 = Bundle("Atom Name"=w86, "Output Array"=w85) -> (w84:T4)  [unwired: 1 in]
          }
        }
      }
    }
    frame True {
      # "Atom array are sorted by distance"
    }
  }
  "Supercell without slab" <- w3
  "Slab" <- w4
  n43 = Index Array(array=w4) -> (element=w10:cluster{"Atom Name":string, "Array":dbl[][]})  [unwired: 1 in]
  n44 = Index Array(array=w3) -> (element=w12:cluster{"Atom Name":string, "Array":dbl[][]})  [unwired: 1 in]
  n45 = Unbundle By Name(w10) -> ("Array"=w11:dbl[][])
  n46 = Unbundle By Name(w12) -> ("Array"=w1:dbl[][])
  n47 = Index Array(array=w11, index (row)=0) -> (element=w2:dbl[])  [unwired: 1 in]
  n48 = stacked-sequence {
    tunnel: w4 -> [w108]
    tunnel: w3 -> [w107]
    tunnel: w1 -> [w106]
    tunnel: w2 -> [w105]
    frame #0 {
      n49 = Delete From Array(array=w105, index="X index to Search") -> (deleted portion=w112:dbl, array with subset deleted=w109:dbl[])  [unwired: 1 in]
      n50 = for {
        tunnel: w106 -> [w160] mode=indexing
        tunnel: w109 -> [w161]
        shift-right: [w159] -> _
        shift-left: dbl[][] [] -> [w158]
        shift-right: [w157] -> w99
        shift-left: dbl[] [] -> [w156]
        tunnel: w112 -> [w155]
        shift-right: [w151] -> _
        shift-left: i32[] [] -> [w150]
        tunnel: "X index to Search" -> [w148]
        tunnel: [w146] -> w101 mode=indexing
        tunnel: [w142] -> w100 mode=indexing
        i -> [w152]
        n51 = Delete From Array(array=w160, index=w148) -> (deleted portion=w154:dbl, array with subset deleted=w146:dbl[])  [unwired: 1 in]
        n52 = Subtract(x=w161, y=w146) -> (x-y=w145:dbl[])
        n53 = local read "Tolerance (A)"() -> (w149:dbl)
        n54 = Subtract(x=w154, y=w155) -> (x-y=w153:dbl)
        n55 = Square(x=w145) -> (x^2=w144:dbl[])
        n56 = Add Array Elements(numeric array=w144) -> (sum=w143:dbl)
        n57 = Square Root(x=w143) -> (sqrt(x)=w142:dbl)
        n58 = Less Or Equal?(x=w142, y=w149) -> (x <= y?=w147:bool)
        n59 = case shown="False" w147 {
          tunnel: w160 -> [_ w173]
          tunnel: [w164 w172] -> w159
          tunnel: w158 -> [w164 w171]
          tunnel: w153 -> [_ w170]
          tunnel: [w163 w169] -> w157
          tunnel: w156 -> [w163 w168]
          tunnel: w152 -> [_ w167]
          tunnel: [w162 w166] -> w151
          tunnel: w150 -> [w162 w165]
          frame False {
          }
          frame True {
            n60 = Build Array (concatenate)(w165, w167) -> (w166:i32[])
            n61 = Build Array (concatenate)(w168, w170) -> (w169:dbl[])
            n62 = Build Array (concatenate)(w171, w173) -> (w172:dbl[][])
          }
        }
      }
      "Array 2" <- w101
      "Array 3" <- w100
      n63 = Sort 1D Array(array=w99) -> (sorted array=w98:dbl[])
      "Length Candidates X" <- w98
      n64 = for {
        tunnel: w98 -> [w116] mode=indexing
        tunnel: w108 -> [w118]
        tunnel: w107 -> [w117]
        tunnel: [w116] -> w104
        tunnel: "X index to Search" -> [w115]
        tunnel: [w114] -> w102
        stop <- w114 stop-if-true
        n65 = for {
          tunnel: w118 -> [w125] mode=indexing
          tunnel: w117 -> [w124] mode=indexing
          tunnel: [w121] -> w114
          tunnel: w116 -> [w120]
          tunnel: w115 -> [w119]
          stop <- w121 continue-if-true
          n66 = Unbundle By Name(w125) -> ("Array"=w123:dbl[][])
          n67 = Unbundle By Name(w124) -> ("Array"=w122:dbl[][])
          n68 = for {
            tunnel: w123 -> [w132] mode=indexing
            tunnel: w122 -> [w129]
            tunnel: [w127] -> w121
            tunnel: w120 -> [w128]
            tunnel: w119 -> [w126]
            stop <- w127 continue-if-true
            n69 = Index Array(array=w132, index=w126) -> (element=w133:dbl)
            n70 = Add(x=w133, y=w128) -> (x+y=w131:dbl)
            n71 = Replace Array Subset(array=w132, new element=w131, index=w126) -> (w130:dbl[])
            n72 = for {
              tunnel: w130 -> [w141]
              tunnel: w129 -> [w140] mode=indexing
              tunnel: [w138] -> w127
              stop <- w138 stop-if-true
              # "Compare offset slabs to supercell"
              n73 = Subtract(x=w141, y=w140) -> (x-y=w135:dbl[])
              n74 = local read "Tolerance (A)"() -> (w139:dbl)
              n75 = Square(x=w135) -> (x^2=w136:dbl[])
              n76 = Add Array Elements(numeric array=w136) -> (sum=w137:dbl)
              n77 = Square Root(x=w137) -> (sqrt(x)=w134:dbl)
              n78 = Less Or Equal?(x=w134, y=w139) -> (x <= y?=w138:bool)
            }
          }
        }
      }
      "Repeating X Length Scale" <- w104
      "Subset X found?!" <- w102
    }
  }
  n79 = stacked-sequence {
    tunnel: w4 -> [w182]
    tunnel: w3 -> [w181]
    tunnel: w1 -> [w180]
    tunnel: w2 -> [w179]
    frame #0 {
      n80 = Delete From Array(array=w179, index="Y index to Search") -> (deleted portion=w185:dbl, array with subset deleted=w188:dbl[])  [unwired: 1 in]
      "array w/ subset deleted" <- w188
      n81 = for {
        tunnel: w180 -> [w235] mode=indexing
        tunnel: w188 -> [w236]
        shift-right: [w234] -> _
        shift-left: dbl[][] [] -> [w233]
        shift-right: [w232] -> w176
        shift-left: dbl[] [] -> [w231]
        tunnel: w185 -> [w230]
        shift-right: [w226] -> _
        shift-left: i32[] [] -> [w225]
        tunnel: "Y index to Search" -> [w223]
        tunnel: [w222] -> w177 mode=indexing
        i -> [w227]
        n82 = Delete From Array(array=w235, index=w223) -> (deleted portion=w229:dbl, array with subset deleted=w222:dbl[])  [unwired: 1 in]
        n83 = Subtract(x=w236, y=w222) -> (x-y=w218:dbl[])
        n84 = Subtract(x=w229, y=w230) -> (x-y=w228:dbl)
        n85 = Square(x=w218) -> (x^2=w219:dbl[])
        n86 = Add Array Elements(numeric array=w219) -> (sum=w220:dbl)
        n87 = Square Root(x=w220) -> (sqrt(x)=w217:dbl)
        n88 = Less Or Equal?(x=w217, y="Tolerance (A)") -> (x <= y?=w221:bool)
        n89 = case shown="True" w221 {
          tunnel: w235 -> [_ w248]
          tunnel: [w239 w247] -> w234
          tunnel: w233 -> [w239 w246]
          tunnel: w228 -> [_ w245]
          tunnel: [w238 w244] -> w232
          tunnel: w231 -> [w238 w243]
          tunnel: w227 -> [_ w242]
          tunnel: [w237 w241] -> w226
          tunnel: w225 -> [w237 w240]
          frame False {
          }
          frame True {
            n90 = Build Array (concatenate)(w240, w242) -> (w241:i32[])
            n91 = Build Array (concatenate)(w246, w248) -> (w247:dbl[][])
            n92 = Build Array (concatenate)(w243, w245) -> (w244:dbl[])
          }
        }
      }
      "Array" <- w177
      n93 = Sort 1D Array(array=w176) -> (sorted array=w175:dbl[])
      "Length Candidates Y" <- w175
      n94 = for {
        tunnel: w175 -> [w191] mode=indexing
        tunnel: w182 -> [w193]
        tunnel: w181 -> [w192]
        tunnel: [w191] -> w183
        tunnel: "Y index to Search" -> [w190]
        tunnel: [w189] -> w174
        stop <- w189 stop-if-true
        n95 = for {
          tunnel: w193 -> [w200] mode=indexing
          tunnel: w192 -> [w199] mode=indexing
          tunnel: [w196] -> w189
          tunnel: w191 -> [w195]
          tunnel: w190 -> [w194]
          stop <- w196 continue-if-true
          n96 = Unbundle By Name(w200) -> ("Array"=w198:dbl[][])
          n97 = Unbundle By Name(w199) -> ("Array"=w197:dbl[][])
          n98 = for {
            tunnel: w198 -> [w207] mode=indexing
            tunnel: w197 -> [w204]
            tunnel: [w202] -> w196
            tunnel: w195 -> [w203]
            tunnel: w194 -> [w201]
            stop <- w202 continue-if-true
            n99 = Index Array(array=w207, index=w201) -> (element=w208:dbl)
            n100 = Add(x=w208, y=w203) -> (x+y=w206:dbl)
            n101 = Replace Array Subset(array=w207, new element=w206, index=w201) -> (w205:dbl[])
            n102 = for {
              tunnel: w205 -> [w216]
              tunnel: w204 -> [w215] mode=indexing
              tunnel: [w213] -> w202
              stop <- w213 stop-if-true
              # "Compare offset slabs to supercell"
              n103 = Subtract(x=w216, y=w215) -> (x-y=w210:dbl[])
              n104 = local read "Tolerance (A)"() -> (w214:dbl)
              n105 = Square(x=w210) -> (x^2=w212:dbl[])
              n106 = Add Array Elements(numeric array=w212) -> (sum=w211:dbl)
              n107 = Square Root(x=w211) -> (sqrt(x)=w209:dbl)
              n108 = Less Or Equal?(x=w209, y=w214) -> (x <= y?=w213:bool)
            }
          }
        }
      }
      "Repeating Y Length Scale" <- w183
      "Subset Y found?!" <- w174
    }
  }
